vi "Get Project Ref and Name.vi"(10 "Project Name Selection":string, 11 "ProjectIn":T1) -> (3 "Project out":T1)   [LabVIEW 2020, in "Dashboard.lvlib"]
uses:
  Dashboard.lvlib
  Project Name and Ref--cluster.ctl
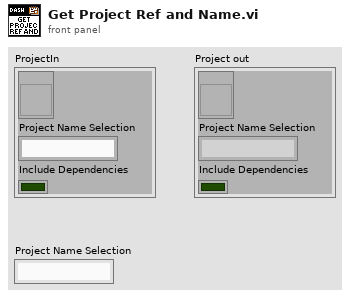
[diagram p1: front panel]
types:
  T1 = typedef "Dashboard.lvlib/Project Name and Ref--cluster.ctl" = cluster{"Project Ref":refnum<vi>, "Project Name Selection":string, "Include Dependencies":bool}
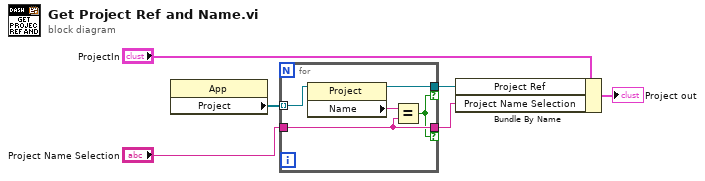
[diagram p0: block diagram]
diagram:
  n1 = property class="App"() -> ("Project"=w5:refnum<vi>[])  [unwired: 2 in, 2 out]
  n2 = for {
    tunnel: w5 -> [w11] mode=indexing
    tunnel: "Project Name Selection" -> [w8]
    tunnel: [w10] -> w4 if=w7
    tunnel: [w8] -> w3 if=w7
    n3 = property class="Project"(reference=w11) -> (reference out=w10:refnum<vi>, "Name"=w9:string)  [unwired: 1 in, 1 out]
    n4 = Equal?(x=w9, y=w8) -> (x = y?=w7:bool)
  }
  n5 = Bundle By Name(cluster="ProjectIn", "Project Ref"=w4, "Project Name Selection"=w3) -> (→"Project out":T1)
